vi "Duplicate.vi"(8 "error in":errorcluster, 10 "parameters":variant, 11 "group in":refnum<class "Group.lvclass">) -> (0 "error out":errorcluster, 3 "group copy":refnum<class "Group.lvclass">)   [LabVIEW 2013, in "Group.lvclass"]
uses:
  Group.lvclass
  Group.lvclass/Group.ctl
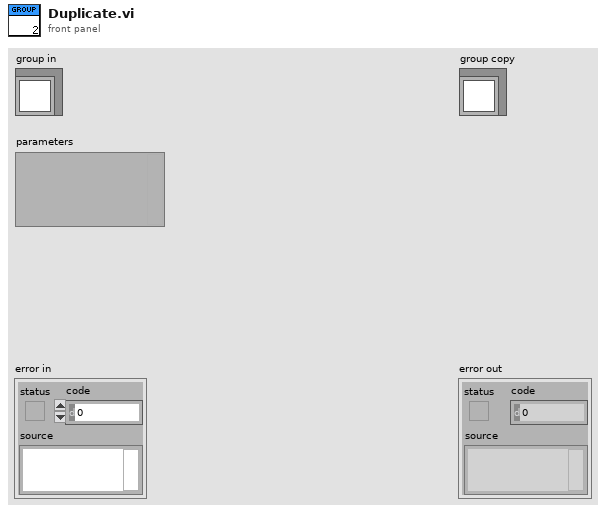
[diagram p1: front panel]
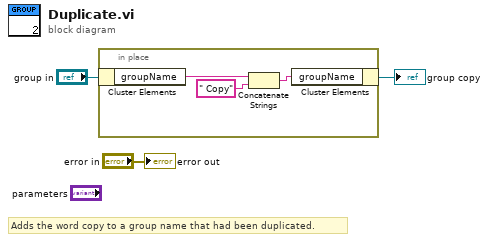
[diagram p0: block diagram]
diagram:
  # "Adds the word copy to a group name that had been duplicated."
  n1 = in-place {
    n2 = in-place-cluster #1("group in") -> ("groupName"=w6:string)
    n3 = Concatenate Strings(w6, " Copy" ("string")) -> (w4:string)
    n4 = in-place-cluster #1("groupName"=w4) -> (→"group copy":refnum<class "Group.lvclass">)
  }
  "error out" <- "error in"
